vi "SetLineFrequency.vi"(8 "Error In":errorcluster, 9 "Line Frequency [50*,60]":T1, 11 "Keithley 6482 In":refnum<visa-resource-name>) -> (0 "Error Out":errorcluster, 3 "Keithley 6482 Out":refnum<visa-resource-name>)   [LabVIEW 2014, in "Keithley-6482-Visa.lvlib"]
uses:
  Keithley-6482-Visa.lvlib
  Controls/LineFrequencyEnum.ctl
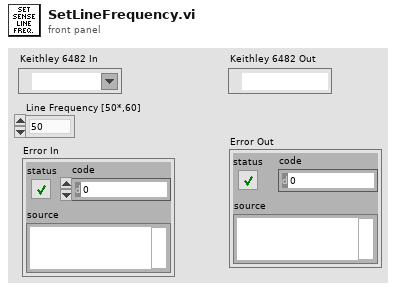
[diagram p1: front panel]
types:
  T1 = typedef "Keithley-6482-Visa.lvlib/LineFrequencyEnum.ctl" = enum16{"50", "60"}
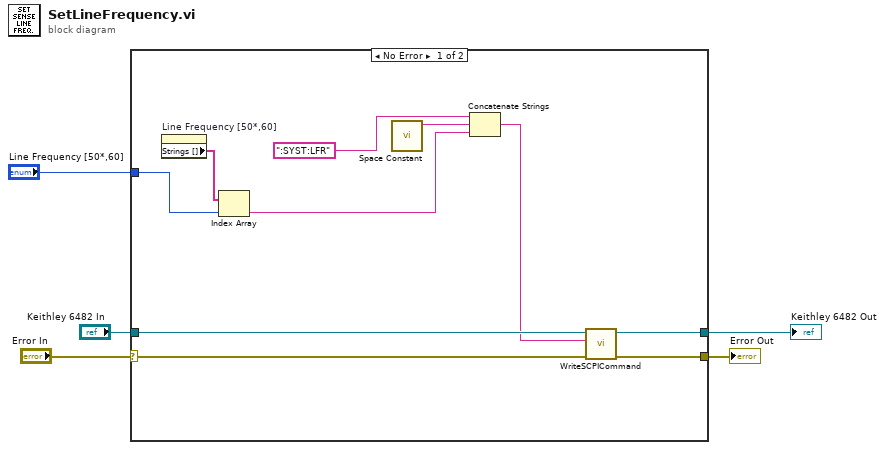
[diagram p0: block diagram]
diagram:
  n1 = case shown="No Error" "Error In" {
    selector: "Error In" -> [w15 w16]
    tunnel: "Keithley 6482 In" -> [w14 w17]
    tunnel: [w9 w16] -> w3
    tunnel: [w10 w17] -> w2
    tunnel: "Line Frequency [50*,60]" -> [w8 _]
    frame No Error {
      n2 = property on="Line Frequency [50*,60]" class="Enum (strict)"() -> ("Strings []"=w6:string[])  [unwired: 2 in, 2 out]
      n3 = Index Array(array=w6, index=w8) -> (element=w7:string)
      n4 = call <vilib>:"Space Constant.vi"() -> ("String"=w12:string)
      n5 = Concatenate Strings(":SYST:LFR" ("string"), w12, w7) -> (w11:string)
      n6 = call "WriteSCPICommand.vi"("Error In"=w15, "SCPI Command"=w11, "Keithley 6482 In"=w14) -> ("Error Out"=w9:errorcluster, "Keithley 6482 Out"=w10:refnum<visa-resource-name>)  [unwired: 7 in]
    }
    frame Error {
    }
  }
  "Error Out" <- w3
  "Keithley 6482 Out" <- w2
